vi "LiveImage_Global.vi"() -> ()   [LabVIEW 2015]
panel:
  out "Max X Pixels":i32=512
  out "Max Y Pixels":i32=512
  out "vmax":i32=512
  out "vmin":i32=1
  out "hmax":i32=512
  out "hmin":i32=1
  out "ImgData":u16[](array[numeric])
  out "Intensity Graph Alt":i32[][](graph)
  in  "Exposure Time":dbl=50.0
  out "ypixels":i32=512
  out "xpixels":i32=512
  out "Intensity Graph":i32[][](graph)
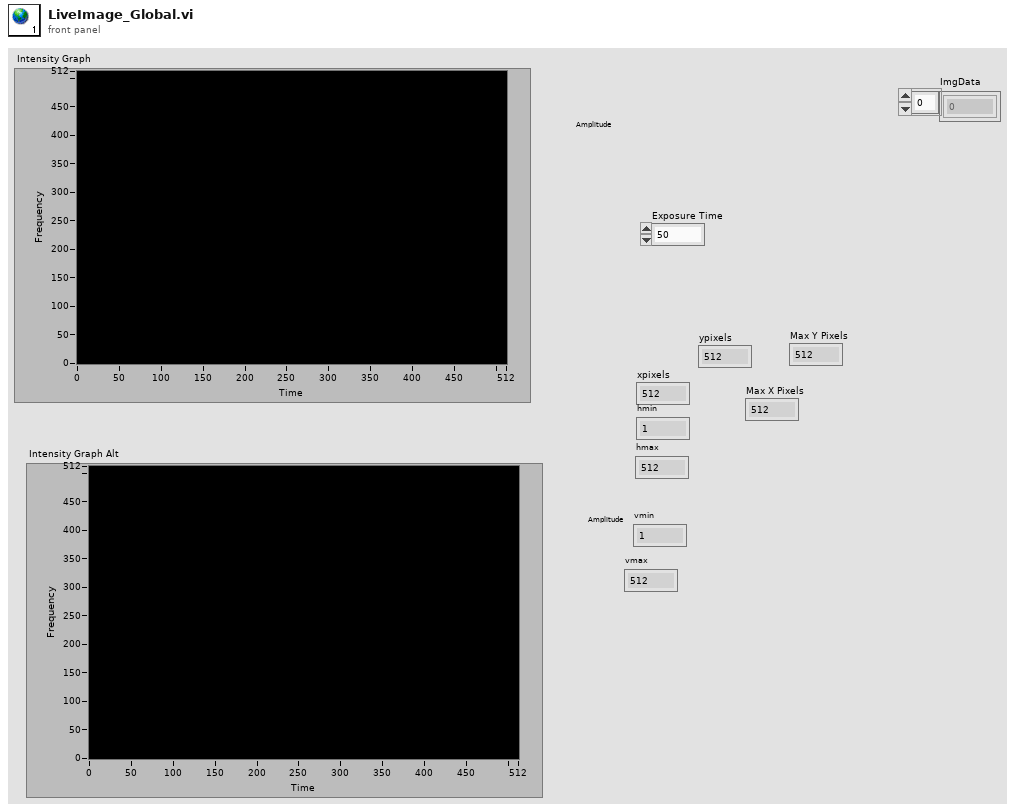
[diagram p1: front panel]
diagram:
